vi "Arrays.vi"(8 "Error In":errorcluster, 11 "ByteBuffer In":refnum<class "ByteBuffer.lvclass">) -> (0 "Error Out":errorcluster, 2 "Arrays":u8[](array[numeric]), 3 "ByteBuffer Out":refnum<class "ByteBuffer.lvclass">, 4 "Has Arrays":bool)   [LabVIEW 2015, in "ByteBuffer.lvclass"]
doc: "Returns the array that backs this buffer.\nThis method is intended to allow array-backed buffers to be passed to native code more efficiently. Concrete subclasses provide more strongly-typed return values for this method.\nModifications to this buffer's content will cause the returned array's content to be modified, and vice versa.\n\nReturns:\nThe array that backs this buffer."
uses:
  ByteBuffer.lvclass
  ByteBuffer.lvclass/ByteBuffer.ctl
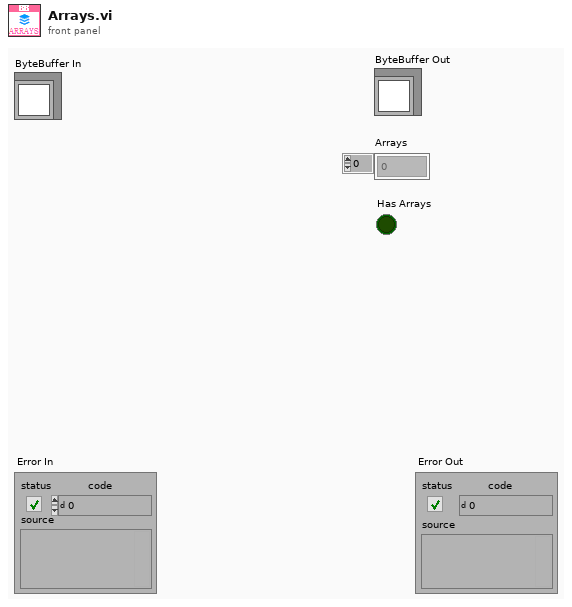
[diagram p1: front panel]
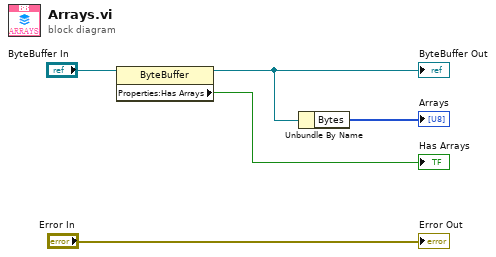
[diagram p0: block diagram]
diagram:
  n1 = property class="ByteBuffer"(reference="ByteBuffer In") -> (reference out=w3:refnum<class "ByteBuffer.lvclass">, "Properties:Has Arrays"=→"Has Arrays":bool)  [unwired: 1 in, 1 out]
  "ByteBuffer Out" <- w3
  n2 = Unbundle By Name(w3) -> ("Bytes"=→"Arrays":u8[])
  "Error Out" <- "Error In"
